vi "Return Data Format.vi"(10 "String In":string) -> (1 "Bytes of Each Point":u8, 2 "Data Format":u16(ring) items=["Byte", "Word"])   [LabVIEW 2020, in "Agilent 90000 Series.lvlib"]
doc: "Returns the data format configuration by the string queried from the instrument."
uses:
  Agilent 90000 Series.lvlib
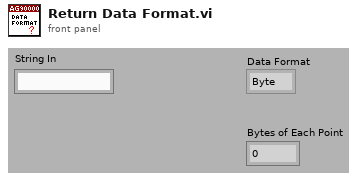
[diagram p1: front panel]
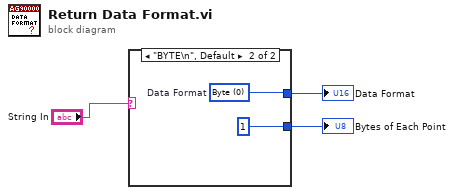
[diagram p0: block diagram]
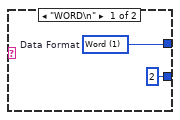
[diagram p2: hidden frame]
diagram:
  n1 = case shown="\"BYTE\\n\", Default" "String In" {
    tunnel: [u8 2 u8 1] -> w2
    tunnel: [w4 w7] -> w1
    frame "WORD\n" {
      w4 = u16 1 items=["Byte", "Word", "Others"]  # Data Format
    }
    frame "BYTE\n", Default {
      w7 = u16 0 items=["Byte", "Word", "Others"]  # Data Format
    }
  }
  "Bytes of Each Point" <- w2
  "Data Format" <- w1
